vi "Button Press.vi"(11 "Button":bool) -> (3 "Button Pressed?":bool)   [LabVIEW 2019]
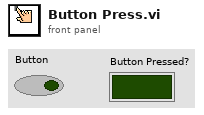
[diagram p1: front panel]
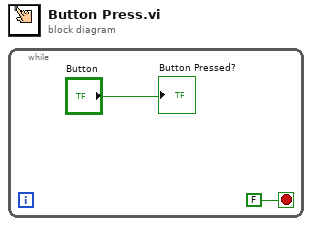
[diagram p0: block diagram]
diagram:
  n1 = while {
    stop <- FALSE stop-if-true
    "Button Pressed?" <- "Button"
  }
